vi "Example Graph - Intensity Callback.vi"(4 "Intensity":refnum<user-event>, 5 "Event Data":cluster{"sender":refnum<k24>, "intensity":i32}, 6 "Control Ref":refnum<k24>, 7 "Event Common Data":T1) -> ()   [LabVIEW 2010]
uses:
  C:/tf/play/labview/Tinkerforge.dll
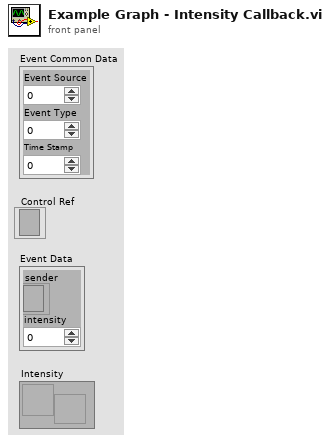
[diagram p1: front panel]
types:
  T1 = cluster{"Event Source":i32, "Event Type":u32, "Time Stamp":u32}
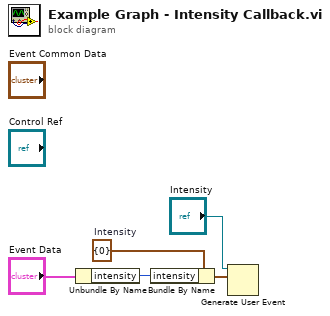
[diagram p0: block diagram]
diagram:
  w3 = cluster{"intensity":i32} {"intensity"=0}  # Intensity
  n1 = Unbundle By Name("Event Data") -> ("intensity"=w4:i32)
  n2 = Bundle By Name(cluster=w3, "intensity"=w4) -> (w2:cluster{"intensity":i32})
  n3 = Generate User Event(user event="Intensity", event data cluster=w2) -> ()  [unwired: 1 in, 2 out]
